vi "niFpgaVivadoProjectExport_Constants.vi"() -> ()   [LabVIEW 2017]
panel:
  out "Pre bitfile tcl filename":string="PreGenerateBitfile.tcl"
  out "Exported files list":string="ExportedFilesList.txt"
  out "LabVIEW folder config key":string="LabVIEWInstallationPath"
  out "Vivado folder config key":string="VivadoDesignSuiteInstallationPath"
  out "Config filename":string="environment.ini"
  out "Vivado log filename":string="VivadoOutput.txt"
  out "Create bitfile utility relative path":path=path "vi.lib/rvi/CDR/createBitfile.exe"
  out "Launch Vivado batch filename":string="LaunchVivadoDesignSuite.bat"
  out "Create bitfile batch filename":string="CreateBitfile.bat"
  out "Project setup tcl filename":string="ProjectSetup.tcl"
  out "Post bitfile tcl filename":string="PostGenerateBitfile.tcl"
  out "Vivado project folder name":string="VivadoProject"
  out "User folder name":string="User"
  out "Protected files folder name":string="NIProtectedFiles"
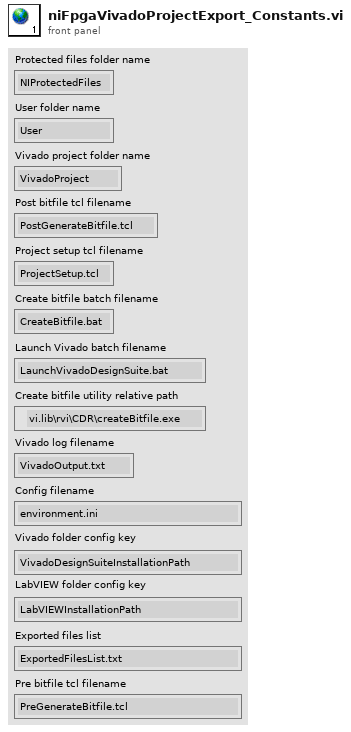
[diagram p1: front panel]
diagram:
